vi "Second Driver.vi"() -> (0 "Second Driver Enabled":bool, 1 "Triggers of Second Controller":cluster{"Left":dbl, "Right":dbl})   [LabVIEW 2015]
uses:
  <vilib>/Rock Robotics/Network Tables/NT Read Number.vi
  Framework/Robot Global Data.vi
  <vilib>/Rock Robotics/WPI/Joystick/WPI_JoystickDeviceEnum.ctl
  Logitech/F510/F510-X.vi
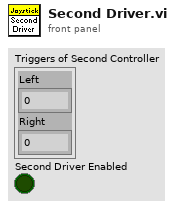
[diagram p1: front panel]
types:
  T1 = typedef "WPI_JoystickDeviceEnum.ctl" = enum16{"USB 0", "USB 1", "USB 2", "USB 3", "USB 4", "USB 5"}
  T2 = typedef "WPI_JoystickDevRef.ctl" = cluster{"Device":T1}
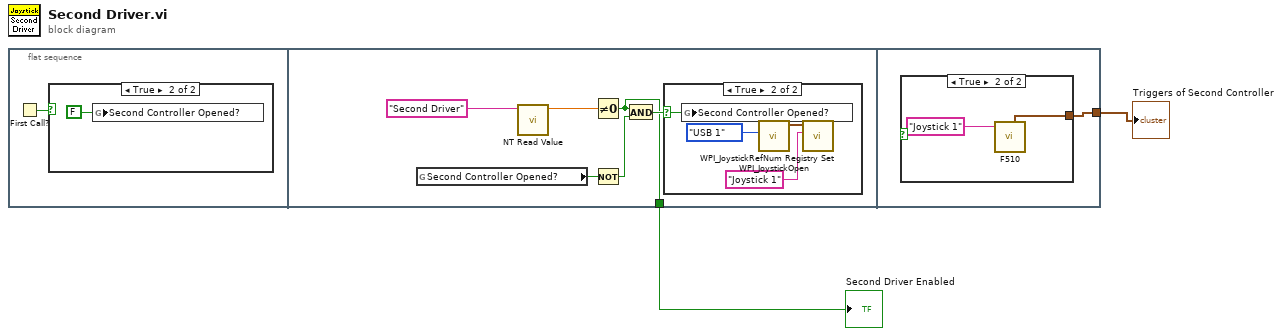
[diagram p0: block diagram]
diagram:
  n1 = flat-sequence {
    tunnel: [w5] -> w1
    tunnel: [w15] -> w2
    frame #0 {
      n2 = First Call?() -> (First Call?: T/F=w3:bool)
      n3 = case shown="True" w3 {
        frame False {
        }
        frame True {
          n4 = global write "Robot Global Data.vi" "Second Controller Opened?"(FALSE) -> ()
        }
      }
    }
    frame #1 {
      n5 = global read "Robot Global Data.vi" "Second Controller Opened?"() -> (w7:bool)
      n6 = call-poly <vilib>:"NT Read Value.vi"("Name"="Second Driver") -> ("Numeric"=w9:dbl)  [unwired: 9 in, 1 out]
      n7 = Not Equal To 0?(x=w9) -> (x != 0?=w5:bool)
      n8 = Not(x=w7) -> (.not. x?=w6:bool)
      n9 = And(x=w5, y=w6) -> (x .and. y?=w8:bool)
      n10 = case shown="True" w8 {
        selector: w8 -> [_ w14]
        frame False {
        }
        frame True {
          n11 = global write "Robot Global Data.vi" "Second Controller Opened?"(w14) -> ()
          n12 = call <vilib>:"WPI_JoystickOpen.vi"("JoystickDevice"=WPI_JoystickDeviceEnum."USB 1") -> ("JoystickDevRef"=w12:T2)  [unwired: 10 in]
          n13 = call <vilib>:"WPI_JoystickRefNum Registry Set.vi"("refnum name"="Joystick 1", "JoystickDevRef"=w12) -> ()  [unwired: 8 in, 2 out]
        }
      }
    }
    frame #2 {
      n14 = case shown="True" {
        selector: _ -> [_ _]
        tunnel: [_ w16] -> w15
        frame False {
        }
        frame True {
          n15 = call-poly "F510.vi"("refnum name"="Joystick 1") -> ("Triggers"=w16:cluster{"Left":dbl, "Right":dbl})  [unwired: 4 in, 6 out]
        }
      }
    }
  }
  "Triggers of Second Controller" <- w2
  "Second Driver Enabled" <- w1
